vi "Remove Observer.vi"(8 "error in (no error)":errorcluster, 10 "Actor Framework.lvlib:Message Enqueuer":refnum<class "Message Enqueuer.lvclass">, 11 "Subject in":refnum<class "Subject.lvclass">) -> (0 "error out":errorcluster, 3 "Subject out":refnum<class "Subject.lvclass">)   [LabVIEW 2013, in "Observer Pattern Actor Interface.lvlib" / "Subject.lvclass"]
uses:
  Subject.lvclass
  <vilib>/ActorFramework/Message Enqueuer/Message Enqueuer.lvclass
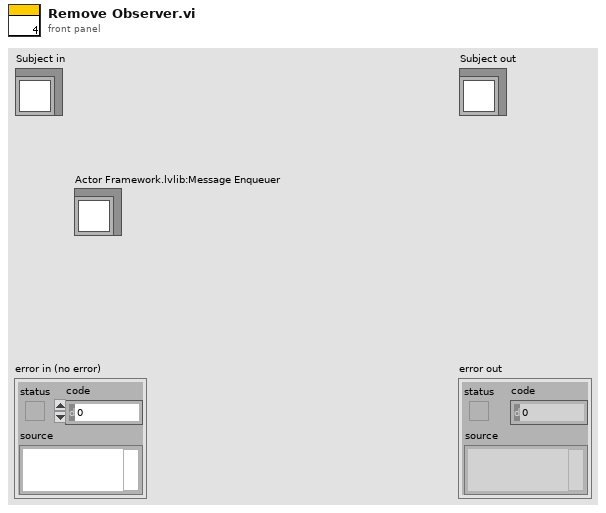
[diagram p1: front panel]
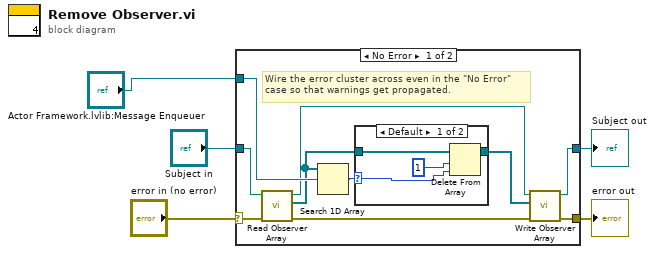
[diagram p0: block diagram]
diagram:
  n1 = case shown="No Error" "error in (no error)" {
    selector: "error in (no error)" -> [w9 w21]
    tunnel: [w8 w21] -> w4
    tunnel: [w11 w20] -> w2
    tunnel: "Subject in" -> [w13 w20]
    tunnel: "Actor Framework.lvlib:Message Enqueuer" -> [w15 _]
    frame No Error {
      # "Wire the error cluster across even in the \"No Error\"\ncase so that warnings get propagated."
      n2 = call "Read Observer Array.vi"("error in (no error)"=w9, "Subject in"=w13) -> ("error out"=w10:errorcluster, "Observer Array"=w6:refnum<class "Message Enqueuer.lvclass">[], "Subject out"=w12:refnum<class "Subject.lvclass">)  [unwired: 7 in]
      n3 = Search 1D Array(1D array=w6, element=w15) -> (index of element=w14:i32)  [unwired: 1 in]
      n4 = case shown="Default" w14 {
        selector: w14 -> [w18 _]
        tunnel: w6 -> [w17 _]
        tunnel: [w16 _] -> w7
        frame Default {
          n5 = Delete From Array(array=w17, length=1, index=w18) -> (array with subset deleted=w16:refnum<class "Message Enqueuer.lvclass">[])  [unwired: 1 out]
        }
        frame -1 {
        }
      }
      n6 = call "Write Observer Array.vi"("error in (no error)"=w10, "Observer Array"=w7, "Subject in"=w12) -> ("error out"=w8:errorcluster, "Subject out"=w11:refnum<class "Subject.lvclass">)  [unwired: 7 in]
    }
    frame Error {
    }
  }
  "error out" <- w4
  "Subject out" <- w2
